vi "op_biti_v1_01.vi"() -> ()   [LabVIEW 2009]
panel:
  in  "Numeric":u8=75
  out "Array":bool[](array[boolean])=[FALSE, TRUE, FALSE, FALSE, TRUE, FALSE, TRUE, TRUE]
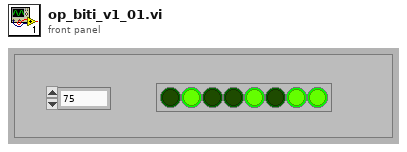
[diagram p1: front panel]
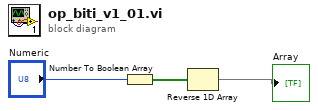
[diagram p0: block diagram]
diagram:
  n1 = Number To Boolean Array(number="Numeric") -> (Boolean array=w3:bool[])
  n2 = Reverse 1D Array(array=w3) -> (reversed array=→"Array":bool[])
